vi "mod_Set Error.vi"(7 "code":i32, 8 "status":bool) -> (0 "error out":errorcluster)   [LabVIEW 2020, in "niAMT.lvlib"]
doc: "Used to facilitate setting error/warning conditions for the modulation toolkit. \nThe convention used by the toolkit for errors/warning is as follows:\n status = True, code < 0, source = something ---> error\n status = False, code > 0, source = something ---> warning\n status = False, code = 0, source = \"\" ---> no error\n\nTo use this VI, simply wire in the boolean to indicate the presence/absence of the condition. The code will indicate whether you're indicating the presence of an error or a warning. \n\nThe VI will add the name of your VI to the source element of the error out cluster."
uses:
  <vilib>/addons/Modulation/niAMT.lvlib
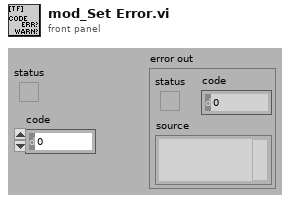
[diagram p1: front panel]
types:
  T1 = cluster{"status":bool, "start index (0)":i32, string}
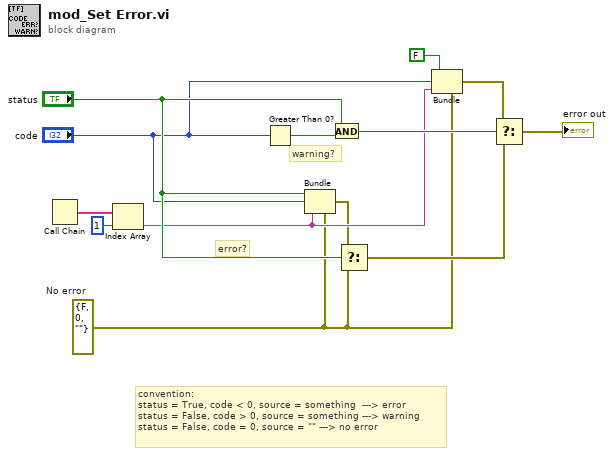
[diagram p0: block diagram]
diagram:
  w2 = T1 {"status"=FALSE, "start index (0)"=0, ""}  # No error
  # "convention:\nstatus = True, code < 0, source = something  ---> error\nstatus = False, code > 0, source = something ---> warning\nstatus = False, code = 0, source = \"\" ---> no error"
  # "error?"
  # "warning?"
  n1 = Call Chain() -> (call chain=w12:string[])
  n2 = Index Array(array=w12, index=1) -> (element=w6:string)
  n3 = Greater Than 0?(x="code") -> (x > 0?=w3:bool)
  n4 = Bundle(cluster=w2, "status"="status", "start index (0)"="code", w6) -> (w5:T1)
  n5 = And(x="status", y=w3) -> (x .and. y?=w9:bool)
  n6 = Select(t=w5, s="status", f=w2) -> (s? t:f=w8:T1)
  n7 = Bundle(cluster=w2, "status"=FALSE, "start index (0)"="code", w6) -> (w11:T1)
  n8 = Select(t=w11, s=w9, f=w8) -> (s? t:f=→"error out":T1)
